vi "Validate Pump Speed.vi"(8 "error in (no error)":errorcluster, 11 "Pump Speed":dbl) -> (0 "error out":errorcluster)   [LabVIEW 2020]
doc: "This example demonstrates how assertation VIs generate and error if the assertation conditions are not met."
uses:
  classes/Assert/Assert.lvclass
panel:
  # "See block diagram"
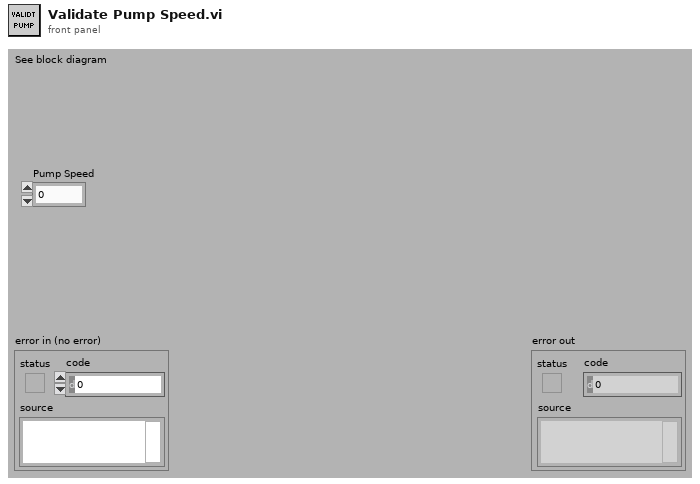
[diagram p1: front panel]
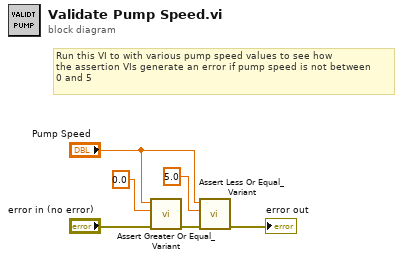
[diagram p0: block diagram]
diagram:
  # "Run this VI to with various pump speed values to see how \nthe assertion VIs generate an error if pump speed is not between\n0 and 5"
  n1 = call "Assert Greater Or Equal_Variant.vi"("error in (no error)"="error in (no error)", "Y"=0.0, "X"="Pump Speed") -> ("error out"=w4:errorcluster)  [unwired: 7 in, 1 out]
  n2 = call "Assert Less Or Equal_Variant.vi"("error in (no error)"=w4, "Y"=5.0, "X"="Pump Speed") -> ("error out"=→"error out":errorcluster)  [unwired: 7 in, 1 out]
